vi "Calibrate_PID.vi"(4 "Which Channel To Control":enum16{"Odor Chan", "Water Chan", "Both"}(ring)=enum."Both", 5 "F1 Stability Threshold":dbl=1.0, 6 "Starting Pressure":dbl[](array[numeric])=[980.7325651117741, 85.55870525881718], 7 "MFCS_EZ":T3=refnum, 8 "Water Mix Pressure Channel":i16=2, 9 "Odor Mix Pressure Channel":i16=1, 10 "Ftot Setpoint":dbl=531.25, 11 "F1 Setpoint":dbl=425.0) -> (2 "Aborted?":bool=TRUE, 3 "Set Pressure Out":dbl[](array[numeric])=[1176.068210890432, 142.32116201879174])   [LabVIEW 2016]
uses:
  <userlib>/Fluigent/Fluigent MFCS/FluigentMFCS_Full.llb/_EZmfcsRefNum.ctl
  <userlib>/Fluigent/Fluigent MFCS/FluigentMFCS_Full.llb/_EZmfcsEnum.ctl
  <vilib>/addons/control/pid/pid.llb/PID Advanced (DBL Array).vi
  <vilib>/addons/control/pid/pid.llb/PID Parameter Manager (DBL Array).vi
  <vilib>/addons/control/pid/pid.llb/PID Derivative Action Buffered (DBL Array).vi
  <vilib>/addons/control/pid/pid.llb/PID Get Advanced Error (DBL Array).vi
  <vilib>/addons/control/pid/pid.llb/PID Integral Action Buffered (DBL Array).vi
  <vilib>/addons/control/pid/pid.llb/PID Resize 1D Array.vi
  <vilib>/addons/control/pid/pid.llb/PID Get Advanced Error (DBL).vi
  Globals/PressuresGlobal.vi
  <vilib>/addons/control/pid/pid.llb/PID Advanced (DBL).vi
  <userlib>/Fluigent/Fluigent MFCS/FluigentMFCS_Full.llb/MFCS_EZ Write Channel Pressure.vi
  <vilib>/addons/control/pid/NI_PID_pid.lvlib
  <vilib>/Analysis/NI_AALBase.lvlib
panel:
  out "PID On":bool=TRUE
  in  "std threshold":dbl=0.15
  out "Var":dbl[](array[numeric])=[7.684799470819524, 0.6885977153199789]
  out "Std":dbl[](array[numeric])=[2.772147086793831, 0.829817880814808]
  in  "Time To Include":dbl=8.0
  out "notification":string="done"
  out "start time":u32=14024200
  out "error out":errorcluster
  in  "Abort":bool
  in  "Tab Control":enum32{"Graph", " Parameters"}(tab)=enum." Parameters"
  out "Stability Progress":u8(slide)=100 scale=0.0..100.0
  out "Error Signal":T1(graph)={"output[0]"=0.034945573808344725, "output[1]"=-0.0056829919234516624, "output[2]"=0.0}
  out "Set Pressure":dbl[](array[numeric])=[1176.068210890432, 142.32116201879174] format="%_10g"
  out "Pressures 2":dbl[](array[numeric])=[1161.0572509765625, 142.331298828125]
  out "Pressures":T2(graph)={"[0]"=1161.0572509765625, "[1]"=142.331298828125, "[2]"=1176.068210890432, "[3]"=142.32116201879174}
  out "Setpoint Reached?":bool
  out "Flow Meter 1 (water flow)":T2(graph)={"[0]"=426.0, "[1]"=424.0, "[2]"=412.5365785212491, "[3]"=425.0}
  out "Flow Meter 2 (total flow)":T2(graph)={"[0]"=531.25, "[1]"=529.4260786657445, "[2]"=531.75, "[3]"=530.75}
  out "Pressure Stable?":bool
  in  "Vals to display":dbl=1235.0
  out "F1":dbl=412.5365785212491
  out "Setpoint":dbl=425.0
  out "F2":dbl=529.4260786657445
  out "Setpoint 2":dbl=531.25
  out "Pressure Channels":i16[](array[numeric])=[2, 1]
  in  "FTot PID gains":cluster{"P":dbl, "I":dbl, "D":dbl}={"P"=0.02, "I"=0.0, "D"=0.0} {"D" format="%.3f"; "I" format="%.3f"; "P" format="%.5f"}
  in  "F1 PID gains":cluster{"P":dbl, "I":dbl, "D":dbl}={"P"=0.004, "I"=0.0, "D"=0.0} {"D" format="%.3f"; "I" format="%.3f"; "P" format="%.5f"}
  in  "linearity":dbl[](array[numeric])=[0.4, 0.4] format="%.2f"
  in  "Ftot Stability Threshold 2":dbl=0.5
  in  "Stable Time (sec)":dbl=10.0
  in  "Total Odor Flow":dbl=425.0
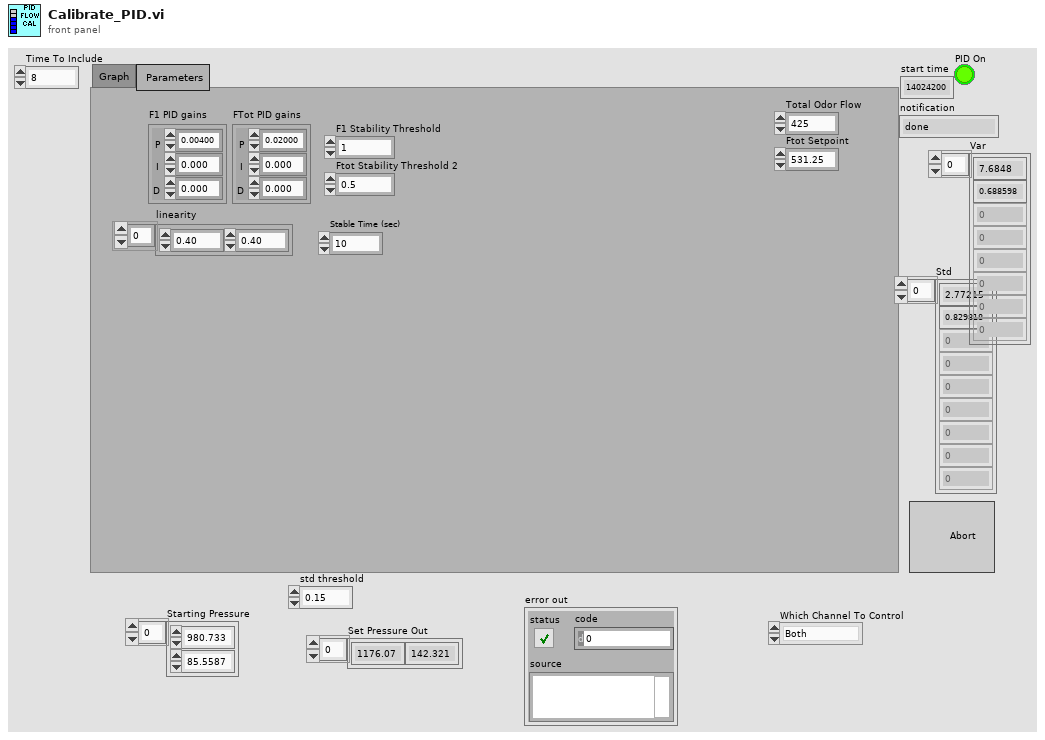
[diagram p1: front panel]
types:
  T1 = cluster{"output[0]":dbl, "output[1]":dbl, "output[2]":dbl}
  T2 = cluster{"[0]":dbl, "[1]":dbl, "[2]":dbl, "[3]":dbl}
  T3 = typedef "_EZmfcsRefNum.ctl" = refnum<k1>
  T4 = cluster{"setpoint high":dbl, "setpoint low":dbl}[]
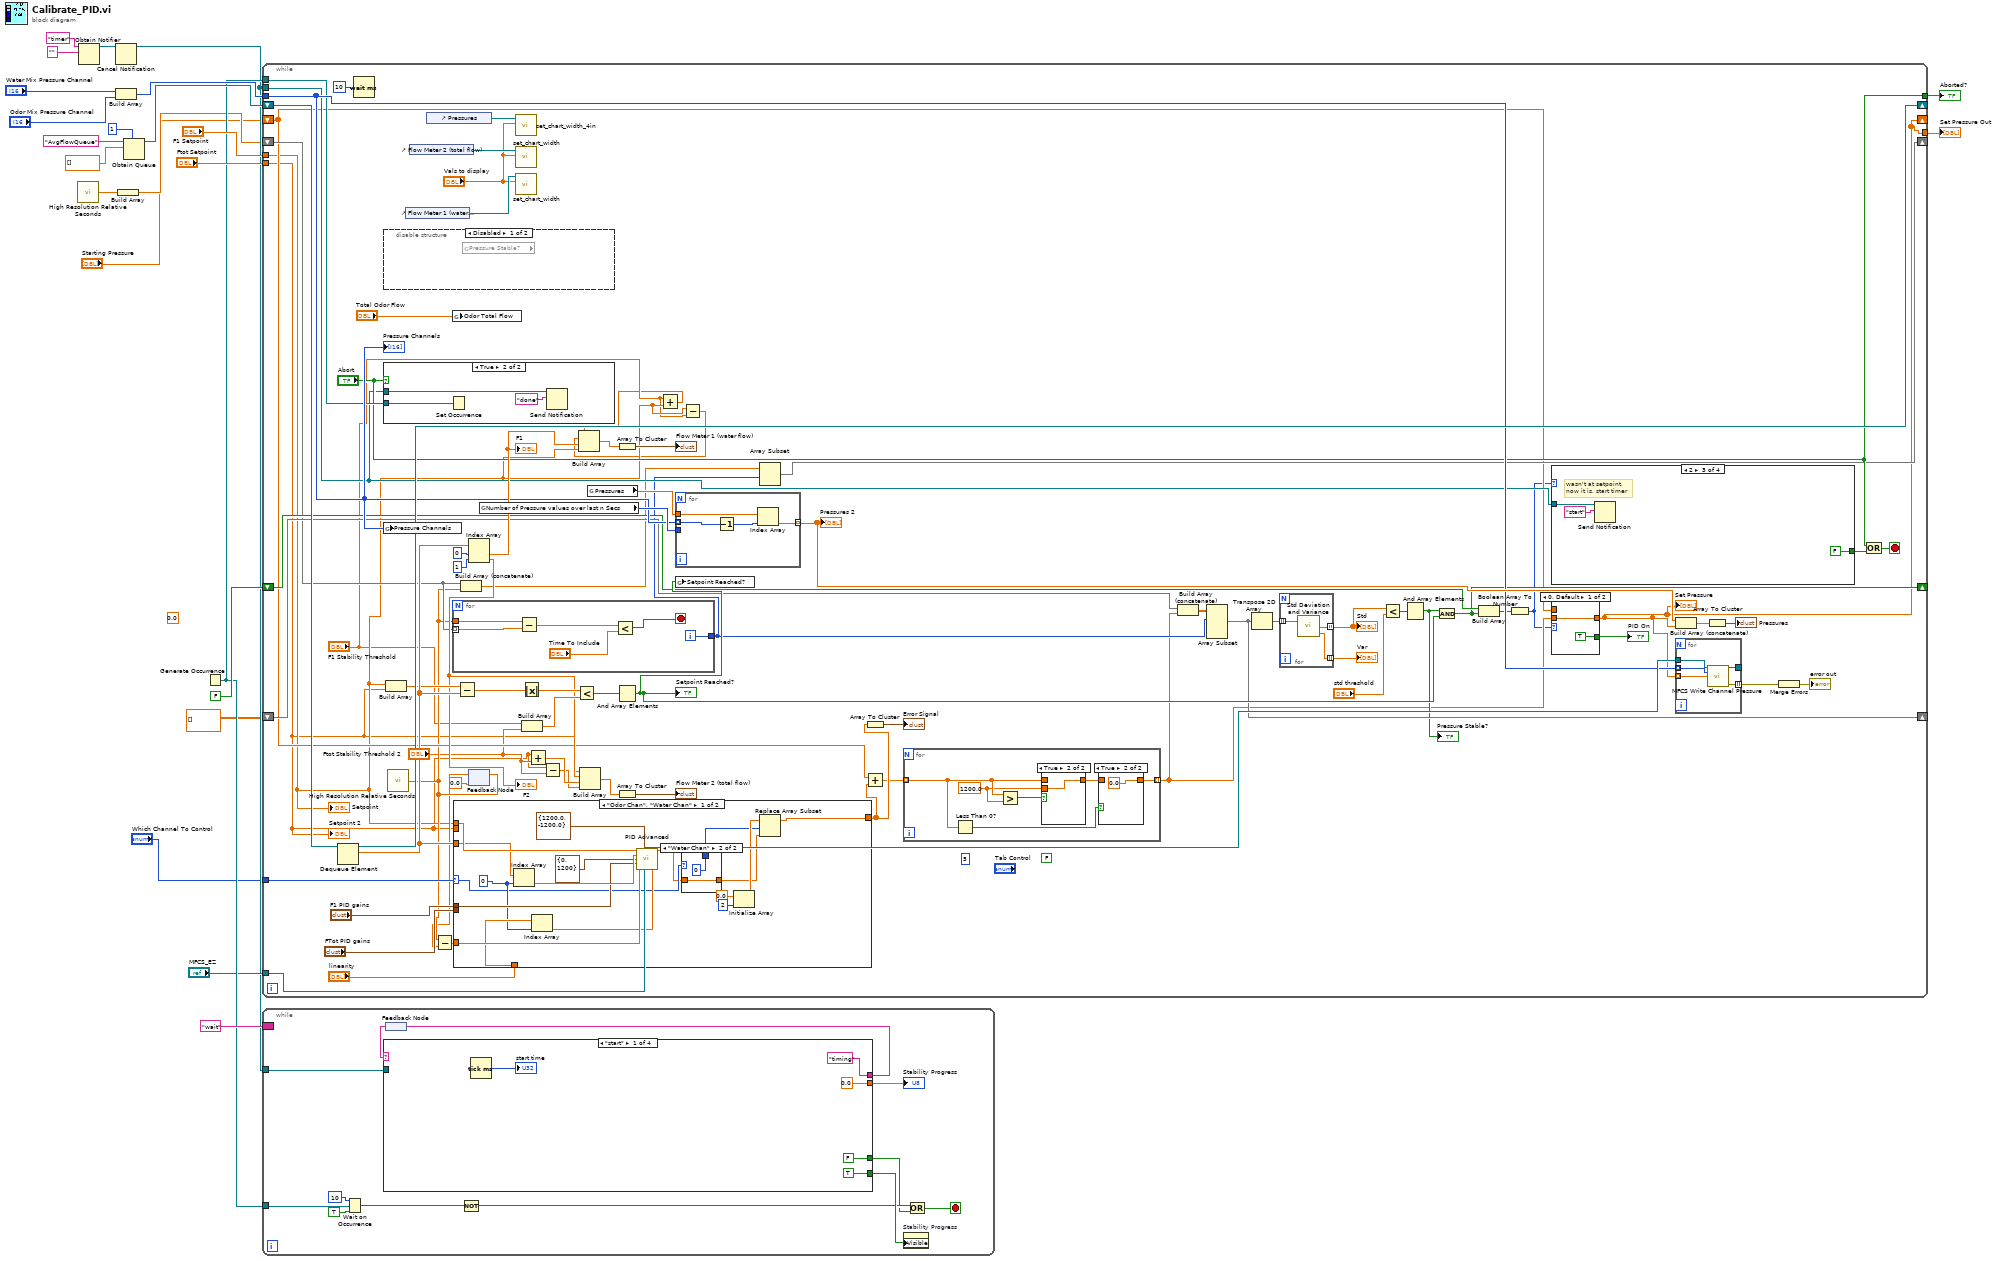
[diagram p0: block diagram]
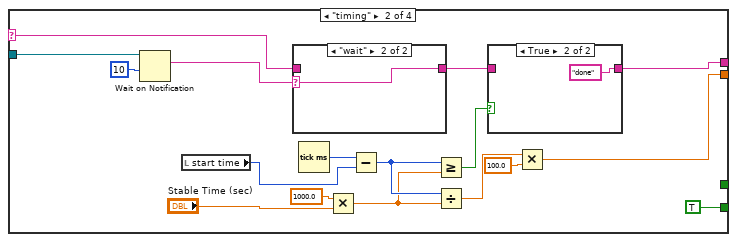
[diagram p2: hidden frame]
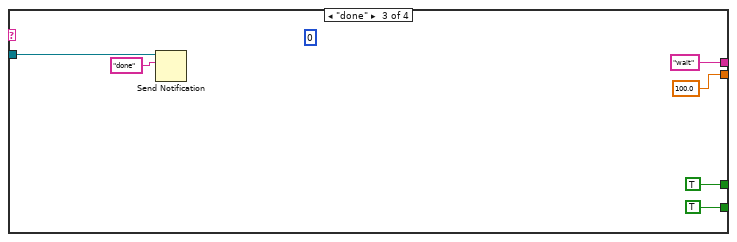
[diagram p5: hidden frame]
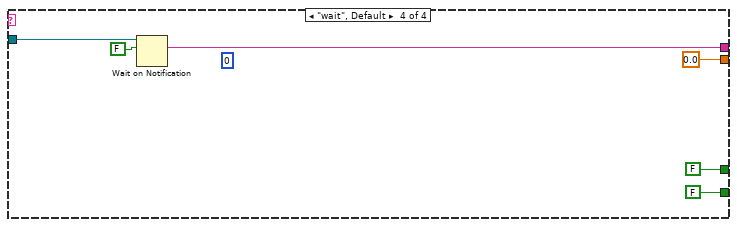
[diagram p6: hidden frame]
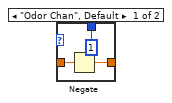
[diagram p7: hidden frame]
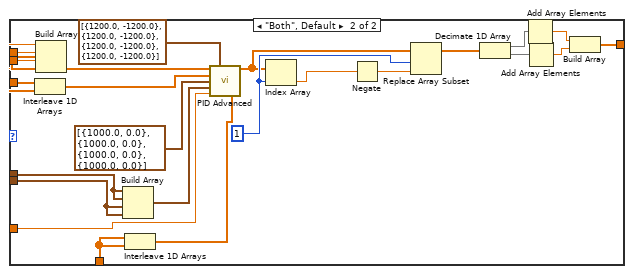
[diagram p8: hidden frame]
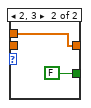
[diagram p9: hidden frame]
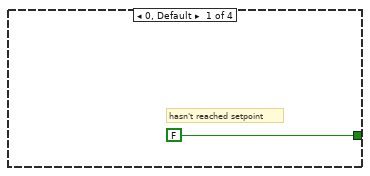
[diagram p14: hidden frame]
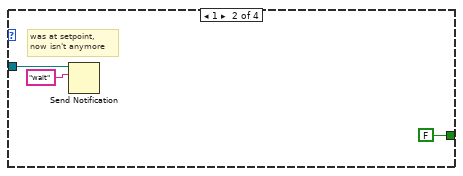
[diagram p15: hidden frame]
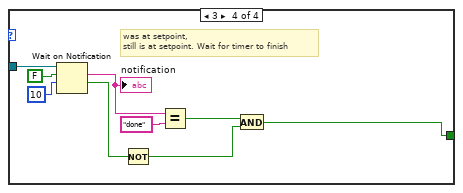
[diagram p16: hidden frame]
diagram:
  (unwired) 0.0 ("array")
  n1 = call <vilib>:"High Resolution Relative Seconds.vi"() -> ("relative seconds"=w4:dbl)
  n2 = Obtain Notifier(name (unnamed)="timer", notification data type="") -> (notifier out=w7:refnum<notifier>)  [unwired: 2 in, 2 out]
  n3 = Cancel Notification(0:w7) -> (8:w6:refnum<notifier>)  [unwired: 1 in, 2 out]
  n4 = Build Array("Water Mix Pressure Channel", "Odor Mix Pressure Channel") -> (w16:i16[])
  n5 = Build Array(w4) -> (w3:dbl[])
  n6 = Obtain Queue(max queue size (-1, unlimited)=1, name (unnamed)="AvgFlowQueue", element data type=dbl[] [] ("appended array")) -> (queue out=w22:refnum<queue>)  [unwired: 2 in, 2 out]
  n7 = Generate Occurrence() -> (w9:refnum<k4>)
  n8 = while {
    shift-right: [w100] -> _
    shift-left: w22 -> [w101]
    tunnel: "MFCS_EZ" -> [w96]
    shift-right: [w40] -> _
    shift-left: "Starting Pressure" -> [w41]
    tunnel: "Ftot Setpoint" -> [w27]
    tunnel: "F1 Setpoint" -> [w32]
    tunnel: w16 -> [w68]
    tunnel: [w40] -> w15
    tunnel: w6 -> [w57]
    shift-right: [w64] -> _
    shift-left: FALSE -> [w65]
    tunnel: ["Abort"] -> w10
    tunnel: w9 -> [w60]
    shift-right: [w48] -> _
    shift-left: dbl[][] [] -> [w54]
    shift-right: [w51] -> _
    shift-left: w3 -> [w50]
    tunnel: "Which Channel To Control" -> [w36]
    stop <- w62 stop-if-true
    (unwired) FALSE
    (unwired) 5
    n9 = Dequeue Element(queue=w101) -> (queue out=w100:refnum<queue>, element=w76:dbl[])  [unwired: 2 in, 2 out]
    n10 = Wait (ms)(milliseconds to wait=u32 10) -> ()  [unwired: 1 out]
    n11 = disable-structure shown="Disabled" {
      frame Disabled {
        n12 = global read "PressuresGlobal.vi" "Pressure Stable?"() -> ()  [unwired: 1 out]
      }
      frame Enabled {
      }
    }
    n13 = case shown="True" "Abort" {
      tunnel: w60 -> [_ w173]
      tunnel: w57 -> [_ w171]
      frame False {
      }
      frame True {
        n14 = Set Occurrence(w173) -> ()
        n15 = Send Notification(notification="done", notifier=w171) -> ()  [unwired: 1 in, 2 out]
      }
    }
    n16 = global write "PressuresGlobal.vi" "Pressure Channels"(w68) -> ()
    n17 = Build Array(w32, w27) -> (w70:dbl[])
    n18 = call <vilib>:"High Resolution Relative Seconds.vi"() -> ("relative seconds"=w35:dbl)
    n19 = control-ref of="Flow Meter 1 (water flow)"() -> (w84:refnum<vi>)
    n20 = control-ref of="Flow Meter 2 (total flow)"() -> (w85:refnum<vi>)
    n21 = control-ref of="Pressures"() -> (w95:refnum<vi>)
    n22 = global write "PressuresGlobal.vi" "Odor Total Flow"("Total Odor Flow") -> ()
    n23 = for {
      tunnel: w35 -> [w157]
      tunnel: w50 -> [w152] mode=indexing
      tunnel: [w154] -> w49
      i -> [w154]
      stop <- w153 stop-if-true
      n24 = Subtract(x=w157, y=w152) -> (x-y=w156:dbl)
      n25 = Less?(x=w156, y="Time To Include") -> (x < y?=w153:bool)
    }
    n26 = Subtract(x=w70, y=w76) -> (x-y=w75:dbl[])
    n27 = Build Array (concatenate)(w50, w35) -> (w52:dbl[])
    n28 = Index Array(array=w76, index #1=0 ("index"), index #2=1 ("index")) -> (element #1=w82:dbl, element #2=w61:dbl)
    "F1" <- w82
    "F2" <- w61
    n29 = feedback #1(0.0 ("relative seconds")) -> (w34:dbl)
    n30 = Subtract(x=w35, y=w34) -> (x-y=w33:dbl)
    n31 = case shown="\"Odor Chan\", \"Water Chan\"" w36 {
      selector: w36 -> [w105 _]
      tunnel: [w106 w133] -> w93
      tunnel: "F1 PID gains" -> [w114 w132]
      tunnel: "FTot PID gains" -> [_ w131]
      tunnel: "linearity" -> [w112 w130]
      tunnel: w76 -> [w118 w128]
      tunnel: w32 -> [w119 w127]
      tunnel: w27 -> [_ w126]
      tunnel: w33 -> [w113 w125]
      frame "Odor Chan", "Water Chan" {
        w110 = 0
        n32 = Index Array(array=w118, index=w110) -> (element=w117:dbl)
        n33 = Index Array(array=w112, index=w110) -> (element=w111:dbl)
        n34 = call-poly <vilib>:"PID Advanced.vi"("setpoint"=w119, "output range"=cluster{"output high":dbl, "output low":dbl} {"output high"=1200.0, "output low"=-1200.0}, "process variable"=w117, "setpoint range"=cluster{"output high":i32, "output low":i32} {"output high"=0, "output low"=1200} ("output range"), "PID gains"=w114, "dt (s)"=w113, "linearity"=w111) -> ("output"=w103:dbl)  [unwired: 7 in, 1 out]
        n35 = case shown="\"Water Chan\"" w105 {
          tunnel: [1 ("dimension size") 0 ("dimension size")] -> w104
          tunnel: w103 -> [w121 w123]
          tunnel: [w120 w123] -> w102
          frame "Odor Chan", Default {
            n36 = Negate(x=w121) -> (-x=w120:dbl)
          }
          frame "Water Chan" {
          }
        }
        n37 = Initialize Array(0.0 ("element"), 2 ("dimension size")) -> (w107:dbl[])
        n38 = Replace Array Subset(array=w107, new element=w102, index=w104) -> (w106:dbl[])
      }
      frame "Both", Default {
        w145 = 1 ("index")
        n39 = Interleave 1D Arrays(w128, w128) -> (w134:dbl[])
        n40 = Build Array(w127, w127, w126, w126) -> (w140:dbl[])
        n41 = Build Array(w132, w132, w131, w131) -> (w141:cluster{"P":dbl, "I":dbl, "D":dbl}[])
        n42 = Interleave 1D Arrays(w130, w130) -> (w129:dbl[])
        n43 = call-poly <vilib>:"PID Advanced.vi"("setpoint"=w140, "output range"=cluster{"output high":dbl, "output low":dbl}[] [{"output high"=1200.0, "output low"=-1200.0}, {"output high"=1200.0, "output low"=-1200.0}, {"output high"=1200.0, "output low"=-1200.0}, {"output high"=1200.0, "output low"=-1200.0}], "process variable"=w134, "setpoint range"=T4 [{"setpoint high"=1000.0, "setpoint low"=0.0}, {"setpoint high"=1000.0, "setpoint low"=0.0}, {"setpoint high"=1000.0, "setpoint low"=0.0}, {"setpoint high"=1000.0, "setpoint low"=0.0}], "PID gains"=w141, "dt (s)"=w125, "linearity"=w129) -> ("output"=w142:dbl[])  [unwired: 7 in, 1 out]
        n44 = Index Array(array=w142, index=w145) -> (element=w144:dbl)
        n45 = Negate(x=w144) -> (-x=w143:dbl)
        n46 = Replace Array Subset(array=w142, new element=w143, index=w145) -> (w139:dbl[])
        n47 = Decimate 1D Array(w139) -> (w138:dbl[], w137:dbl[])
        n48 = Add Array Elements(numeric array=w138) -> (sum=w136:dbl)
        n49 = Add Array Elements(numeric array=w137) -> (sum=w135:dbl)
        n50 = Build Array(w136, w135) -> (w133:dbl[])
      }
    }
    n51 = feedback-in #1(w35) -> ()
    n52 = global read "PressuresGlobal.vi" "Number of Pressure values over last n Secs"() -> (w77:i32[])
    n53 = call "set_chart_width_4in.vi"("Values to Display"="Vals to display", "Ref In"=w95) -> ()  [unwired: 10 in]
    n54 = call "set_chart_width.vi"("Values to Display"="Vals to display", "Ctl Refnum"=w85) -> ()  [unwired: 10 in]
    n55 = call "set_chart_width.vi"("Values to Display"="Vals to display", "Ctl Refnum"=w84) -> ()  [unwired: 10 in]
    n56 = Absolute Value(x=w75) -> (abs(x)=w73:dbl[])
    n57 = Build Array("F1 Stability Threshold", "Ftot Stability Threshold 2") -> (w74:dbl[])
    n58 = Add(x=w27, y="Ftot Stability Threshold 2") -> (x+y=w26:dbl)
    n59 = Subtract(x=w27, y="Ftot Stability Threshold 2") -> (x-y=w25:dbl)
    n60 = Less?(x=w73, y=w74) -> (x < y?=w72:bool[])
    n61 = Build Array(w27, w61, w26, w25) -> (w88:dbl[])
    n62 = global read "PressuresGlobal.vi" "Pressures"() -> (w78:dbl[])
    n63 = And Array Elements(Boolean array=w72) -> (logical AND=w67:bool)
    "Setpoint Reached?" <- w67
    n64 = Array To Cluster(array=w88) -> (cluster=→"Flow Meter 2 (total flow)":T2)
    n65 = Add(x="F1 Stability Threshold", y=w32) -> (x+y=w30:dbl)
    n66 = for {
      tunnel: w68 -> [w192] mode=indexing
      tunnel: w78 -> [w193]
      tunnel: [w191] -> w71 mode=indexing
      tunnel: w77 -> [_]
      n67 = Decrement(x=w192) -> (x-1=w190:i16)
      n68 = Index Array(array=w193, index=w190) -> (element=w191:dbl)
    }
    "Pressures 2" <- w71
    n69 = global write "PressuresGlobal.vi" "Setpoint Reached?"(w67) -> ()
    n70 = Subtract(x=w32, y="F1 Stability Threshold") -> (x-y=w29:dbl)
    n71 = Build Array(w30, w29, w82, w32) -> (w90:dbl[])
    n72 = Array To Cluster(array=w90) -> (cluster=→"Flow Meter 1 (water flow)":T2)
    n73 = Array Subset(array=w52, index=w49) -> (w51:dbl[])  [unwired: 1 in]
    n74 = Array To Cluster(array=w93) -> (cluster=→"Error Signal":cluster{"[0]":dbl, "[1]":dbl, "[2]":dbl})
    n75 = Add(x=w41, y=w93) -> (x+y=w58:dbl[])
    n76 = for {
      tunnel: w58 -> [w162] mode=indexing
      tunnel: [w163] -> w38 mode=indexing
      w161 = 1200.0 ("x")
      n77 = Less Than 0?(x=w162) -> (x < 0?=w164:bool)
      n78 = Greater?(x=w162, y=w161) -> (0:w166:bool)
      n79 = case shown="True" w166 {
        tunnel: [w169 w170] -> w165
        tunnel: w161 -> [_ w170]
        tunnel: w162 -> [w169 _]
        frame False {
        }
        frame True {
        }
      }
      n80 = case shown="True" w164 {
        tunnel: w165 -> [w167 _]
        tunnel: [w167 0.0 ("x")] -> w163
        frame False {
        }
        frame True {
        }
      }
    }
    n81 = Build Array (concatenate)(w54, w38) -> (w53:dbl[][])
    n82 = Array Subset(array=w53, index (row)=w49) -> (w48:dbl[][])  [unwired: 3 in]
    n83 = Transpose 2D Array(2D array=w48) -> (transposed array=w46:dbl[][])
    n84 = for {
      tunnel: w46 -> [w160] mode=indexing
      tunnel: [w159] -> w45 mode=indexing
      tunnel: [w158] -> w47 mode=indexing
      n85 = call <vilib>:"Std Deviation and Variance.vi"("X"=w160) -> ("standard deviation"=w159:dbl, "variance"=w158:dbl)  [unwired: 1 in, 1 out]
    }
    "Var" <- w47
    "Std" <- w45
    n86 = Less?(x=w45, y="std threshold") -> (x < y?=w44:bool[])
    n87 = And Array Elements(Boolean array=w44) -> (logical AND=w43:bool)
    "Pressure Stable?" <- w43
    n88 = And(x=w43, y=w67) -> (x .and. y?=w64:bool)
    n89 = Build Array(w65, w64) -> (w66:bool[])
    n90 = Boolean Array To Number(Boolean array=w66) -> (number=w37:u32)
    n91 = case shown="2" w37 {
      tunnel: w57 -> [_ w176 w180 w189]
      tunnel: [FALSE ("timed out?") FALSE ("timed out?") FALSE ("timed out?") w181] -> w63
      frame 0, Default {
        # "hasn't reached setpoint"
      }
      frame 1 {
        # "was at setpoint, \nnow isn't anymore"
        n92 = Send Notification(notification="wait", notifier=w176) -> ()  [unwired: 1 in, 2 out]
      }
      frame 2 {
        # "wasn't at setpoint,\nnow it is, start timer"
        n93 = Send Notification(notification="start", notifier=w180) -> ()  [unwired: 1 in, 2 out]
      }
      frame 3 {
        # "was at setpoint, \nstill is at setpoint. Wait for timer to finish"
        n94 = Wait on Notification(notifier=w189, ignore previous (F)=FALSE, timeout in ms (-1)=10) -> (notification=w184:string, timed out?=w187:bool)  [unwired: 1 in, 2 out]
        "notification" <- w184
        n95 = Not(x=w187) -> (.not. x?=w182:bool)
        n96 = Equal?(x=w184, y="done" ("notification")) -> (x = y?=w183:bool)
        n97 = And(x=w183, y=w182) -> (x .and. y?=w181:bool)
      }
    }
    n98 = case shown="0, Default" w37 {
      tunnel: w38 -> [w149 _]
      tunnel: w41 -> [_ w151]
      tunnel: [w149 w151] -> w40
      tunnel: [TRUE FALSE] -> w39
      frame 0, Default {
      }
      frame 2, 3 {
      }
    }
    "Set Pressure" <- w40
    "PID On" <- w39
    n99 = for {
      tunnel: [w198] -> _
      tunnel: w68 -> [w197] mode=indexing
      tunnel: w40 -> [w196] mode=indexing
      tunnel: w96 -> [w195]
      tunnel: [w194] -> w55 mode=indexing
      n100 = call-poly <userlib>:"MFCS Write Channel Pressure.vi"("MFCS_EZ"=w195, "Channel Number (default=1)"=w197, "Pressure (mBar)"=w196) -> ("MFCS_EZ out"=w198:T3, "error out"=w194:errorcluster)  [unwired: 11 in]
    }
    n101 = Build Array (concatenate)(w71, w40) -> (w86:dbl[])
    n102 = Array To Cluster(array=w86) -> (cluster=→"Pressures":T2)
    n103 = Merge Errors(w55) -> (→"error out":errorcluster)
    n104 = Or(x="Abort", y=w63) -> (x .or. y?=w62:bool)
    "Setpoint" <- w32
    "Setpoint 2" <- w27
    "Pressure Channels" <- w68
  }
  "Set Pressure Out" <- w15
  "Aborted?" <- w10
  n105 = while {
    tunnel: w6 -> [w210]
    tunnel: w9 -> [w204]
    border: "wait" -> [_]
    stop <- w199 stop-if-true
    n106 = Wait on Occurrence(1:TRUE ("ignore previous (T)"), 2:w204, 3:10 ("ms timeout (-1)")) -> (0:w202:bool)
    n107 = feedback #2() -> (w208:string)
    n108 = case shown="\"start\"" w208 {
      selector: w208 -> [_ w221 _ _]
      tunnel: w210 -> [_ w222 w242 w248]
      tunnel: ["timing" ("notification") w217 "wait" ("notification") w247] -> w209
      tunnel: [FALSE _ TRUE FALSE] -> w200
      tunnel: [0.0 w216 100.0 0.0] -> w207
      tunnel: [TRUE ("Visible") TRUE ("Visible") TRUE ("Visible") FALSE ("Visible")] -> w206
      frame "start" {
        n109 = Tick Count (ms)() -> (millisecond timer value=→"start time":u32)
      }
      frame "timing" {
        n110 = Wait on Notification(notifier=w222, timeout in ms (-1)=10) -> (notification=w231:string)  [unwired: 2 in, 3 out]
        n111 = local read "start time"() -> (w220:u32)
        n112 = case shown="\"wait\"" w231 {
          selector: w231 -> [_ w236]
          tunnel: w221 -> [w235 _]
          tunnel: [w235 w236] -> w227
          frame "start", Default {
          }
          frame "wait" {
          }
        }
        n113 = Tick Count (ms)() -> (millisecond timer value=w219:u32)
        n114 = Multiply(x=1000.0, y="Stable Time (sec)") -> (x*y=w225:dbl)
        n115 = Subtract(x=w219, y=w220) -> (x-y=w226:u32)
        n116 = Greater Or Equal?(x=w226, y=w225) -> (x >= y?=w228:bool)
        n117 = Divide(x=w226, y=w225) -> (x/y=w224:dbl)
        n118 = case shown="True" w228 {
          tunnel: w227 -> [w233 _]
          tunnel: [w233 "done"] -> w217
          frame False {
          }
          frame True {
          }
        }
        n119 = Multiply(x=w224, y=100.0) -> (x*y=w216:dbl)
      }
      frame "done" {
        (unwired) u32 0
        n120 = Send Notification(notification="done", notifier=w242) -> ()  [unwired: 1 in, 2 out]
      }
      frame "wait", Default {
        (unwired) u32 0
        n121 = Wait on Notification(notifier=w248, ignore previous (F)=FALSE) -> (notification=w247:string)  [unwired: 2 in, 3 out]
      }
    }
    "Stability Progress" <- w207
    n122 = feedback-in #2(w209) -> ()
    n123 = Not(x=w202) -> (.not. x?=w201:bool)
    n124 = property on="Stability Progress" class="Slide (strict)"("Visible"=w206) -> ()  [unwired: 2 in, 2 out]
    n125 = Or(x=w201, y=w200) -> (x .or. y?=w199:bool)
  }
